vi "MCP23S17 Out Set.vi"(4 "SW Mode":bool, 6 "Set Single Ch":u16 max=10, 8 "error in (no error)":errorcluster, 9 "Channels":u16 max=1023, 10 "Addr":T1 items=["Addr-0"=0, "Addr-1"=4, "Addr-2"=2, "Addr-3"=6, "Addr-4"=1, "Addr-5"=5, "Addr-6"=3, "Addr-7"=7], 11 "handle":u32 format="%08x") -> (0 "error out":errorcluster, 3 "handle out":u32)   [LabVIEW 2018]
uses:
  PROJEKT/NIKO/Labview/Niko V4/FTDI SPI/Ctl/Sub Addr.ctl
  PROJEKT/NIKO/Labview/Niko V5/FTDI SPI/libMPSSE-SPI.lvlib
panel:
  out "string 4":string
  out "string 3":string
  out "string 2":string
  out "string":string
  in  "Array U8":u8[](array[numeric])=[64, 18, 0, 128, 0, 0, 0, 0, 0, 0] format="%x"
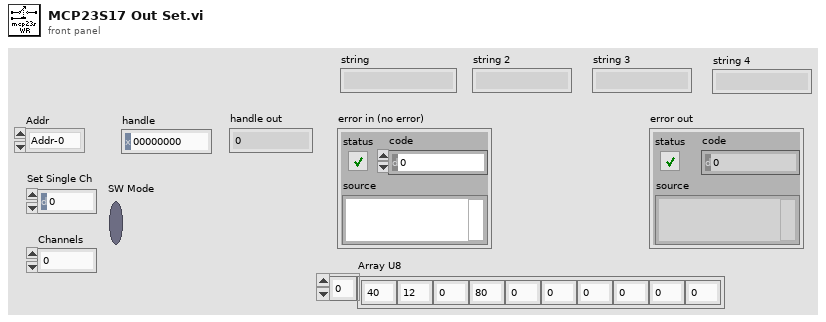
[diagram p1: front panel]
types:
  T1 = typedef "Sub Addr.ctl" = u16
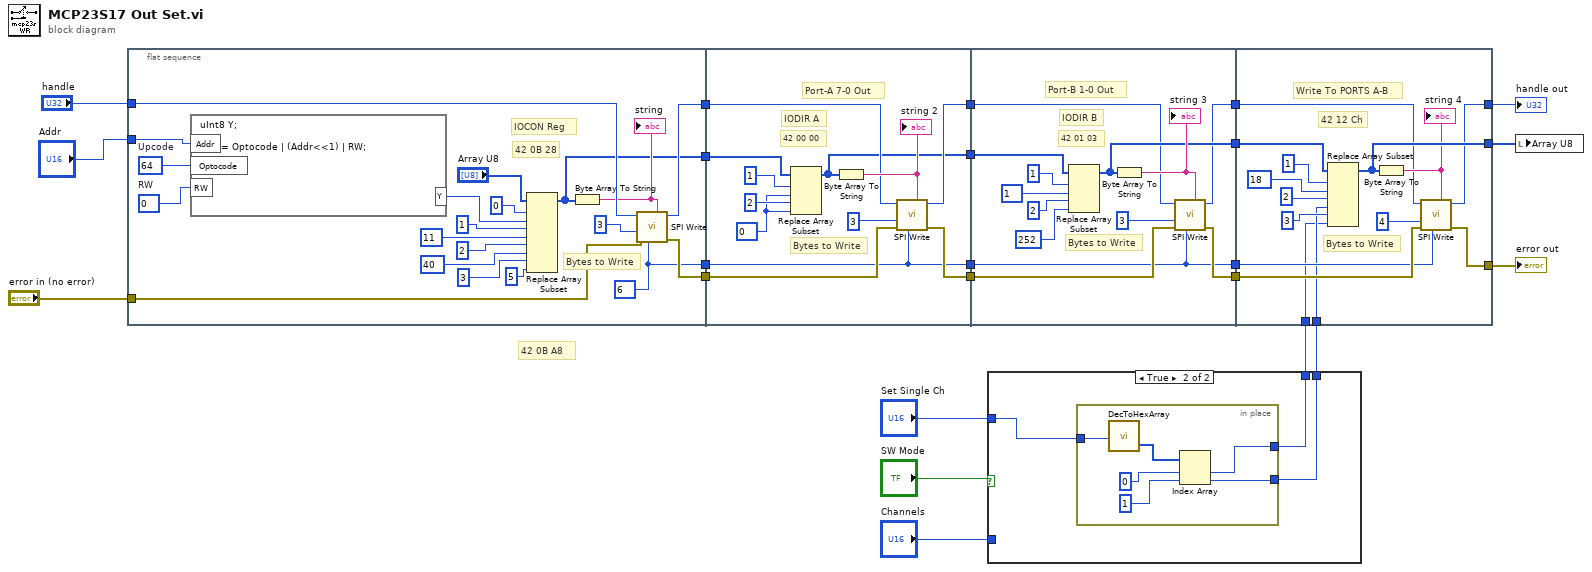
[diagram p0: block diagram]
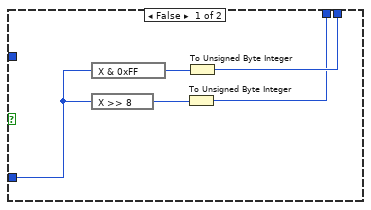
[diagram p2: hidden frame]
diagram:
  # "42 0B A8"
  n1 = flat-sequence {
    tunnel: "Addr" -> [w42]
    tunnel: "handle" -> [w36]
    tunnel: [w34] -> w23
    tunnel: [w33] -> w22
    tunnel: [w32] -> w21
    tunnel: [w31] -> w20
    tunnel: "error in (no error)" -> [w30]
    tunnel: w23 -> [w54]
    tunnel: w22 -> [w48]
    tunnel: w21 -> [w52]
    tunnel: w20 -> [w45]
    tunnel: [w53] -> w19
    tunnel: [w47] -> w18
    tunnel: [w46] -> w17
    tunnel: [w45] -> w16
    tunnel: w19 -> [w63]
    tunnel: w18 -> [w61]
    tunnel: w17 -> [w65]
    tunnel: w16 -> [w56]
    tunnel: [w62] -> w15
    tunnel: [w60] -> w14
    tunnel: [w64] -> w13
    tunnel: [w56] -> w4
    tunnel: [w80] -> w7
    tunnel: [w82] -> w9
    tunnel: [w77] -> w8
    tunnel: w15 -> [w78]
    tunnel: w14 -> [w83]
    tunnel: w13 -> [w81]
    tunnel: w12 -> [w69]
    tunnel: w11 -> [w70]
    tunnel: w4 -> [w71]
    frame #0 {
      w24 = u8 64  # Upcode
      w25 = u8 0  # RW
      w31 = u8 6
      # "IOCON Reg"
      # "Bytes to Write"
      # "42 0B 28"
      n2 = formula code="uInt8 Y;\n      \n    Y = Optocode | (Addr<<1) | RW;"("Addr"=w42, "Optocode"=w24, "RW"=w25) -> ("Y"=w41:u8)
      n3 = Replace Array Subset(array="Array U8", new element #1=w41, index #1=0 ("index"), new element #2=u8 11, index #2=u8 1 ("new element/subarray"), new element #3=u8 40, index #3=2 ("index"), new element #4=u8 5 ("new element/subarray"), index #4=3 ("index")) -> (w32:u8[])
      n4 = Byte Array To String(unsigned byte array=w32) -> (string=w35:string)
      "string" <- w35
      n5 = call "SPI Write.vi"("buffer"=w35, "options"=w31, "error in (no error)"=w30, "Bytes To Send"=u32 3, "handle"=w36) -> ("error out"=w33:errorcluster, "handle out"=w34:u32)  [unwired: 4 in, 1 out]
    }
    frame #1 {
      w49 = u8 0
      # "IODIR A"
      # "Port-A 7-0 Out"
      # "Bytes to Write"
      # "42 00 00"
      n6 = Replace Array Subset(array=w52, new element #1=w49, index #1=1 ("index"), new element #2=w49, index #2=2 ("index")) -> (w46:u8[])
      n7 = Byte Array To String(unsigned byte array=w46) -> (string=w55:string)
      "string 2" <- w55
      n8 = call "SPI Write.vi"("buffer"=w55, "options"=w45, "error in (no error)"=w48, "Bytes To Send"=u32 3, "handle"=w54) -> ("error out"=w47:errorcluster, "handle out"=w53:u32)  [unwired: 4 in, 1 out]
    }
    frame #2 {
      # "IODIR B"
      # "Port-B 1-0 Out"
      # "Bytes to Write"
      # "42 01 03"
      n9 = Replace Array Subset(array=w65, new element #1=u8 1, index #1=1 ("index"), new element #2=u8 252, index #2=2 ("index")) -> (w64:u8[])
      n10 = Byte Array To String(unsigned byte array=w64) -> (string=w66:string)
      "string 3" <- w66
      n11 = call "SPI Write.vi"("buffer"=w66, "options"=w56, "error in (no error)"=w61, "Bytes To Send"=u32 3, "handle"=w63) -> ("error out"=w60:errorcluster, "handle out"=w62:u32)  [unwired: 4 in, 1 out]
    }
    frame #3 {
      # "Write To PORTS A-B"
      # "Bytes to Write"
      # "42 12 Ch"
      n12 = Replace Array Subset(array=w81, new element #1=u8 18, index #1=1 ("index"), new element #2=w70, index #2=2 ("index"), new element #3=w69, index #3=3 ("index")) -> (w80:u8[])
      n13 = Byte Array To String(unsigned byte array=w80) -> (string=w79:string)
      "string 4" <- w79
      n14 = call "SPI Write.vi"("buffer"=w79, "options"=w71, "error in (no error)"=w83, "Bytes To Send"=u32 4, "handle"=w78) -> ("error out"=w82:errorcluster, "handle out"=w77:u32)  [unwired: 4 in, 1 out]
    }
  }
  n15 = case shown="True" "SW Mode" {
    tunnel: [w85 w90] -> w12
    tunnel: [w87 w91] -> w11
    tunnel: "Set Single Ch" -> [_ w89]
    tunnel: "Channels" -> [w84 _]
    frame False {
      n16 = expression code="X & 0xFF"(w84) -> (w88:u16)
      n17 = expression code="X >> 8"(w84) -> (w86:u16)
      n18 = To Unsigned Byte Integer(number=w86) -> (unsigned 8bit integer=w85:u8)
      n19 = To Unsigned Byte Integer(number=w88) -> (unsigned 8bit integer=w87:u8)
    }
    frame True {
      n20 = in-place {
        in-place-border: w89 -> [w92]
        in-place-border: [w96] -> w91
        in-place-border: [w95] -> w90
        n21 = call "DecToHexArray.vi"("Channel To Modify"=w92) -> ("Array HexDec"=w93:u8[])  [unwired: 2 in, 1 out]
        n22 = Index Array(array=w93, index #1=0 ("index"), index #2=1 ("index")) -> (element #1=w95:u8, element #2=w96:u8)
      }
    }
  }
  n23 = local write "Array U8"(w7) -> ()
  "error out" <- w9
  "handle out" <- w8
